vi "Sequence.ConvertColumnHeadersToChannels.vi"(8 "error in (no error)":errorcluster, 9 "Aliases.Outputs":T1[](array[typedef]), 10 "UI.Sequence#ofColumns":i32, 11 "UI.SequenceRef":refnum<vi>) -> (0 "error out":errorcluster, 1 "Warning":string, 3 "Output Channels":T1[](array[typedef]))   [LabVIEW 2015, in "Simple Sequence Tools - Editor.lvlib"]
uses:
  Simple Sequence Tools - Editor.lvlib
  Shared/Types/Channel.Properties.ctl
  Shared/SubVIs/Main.Constants.vi
  Shared/Simple Sequence Tools - Shared.lvlib
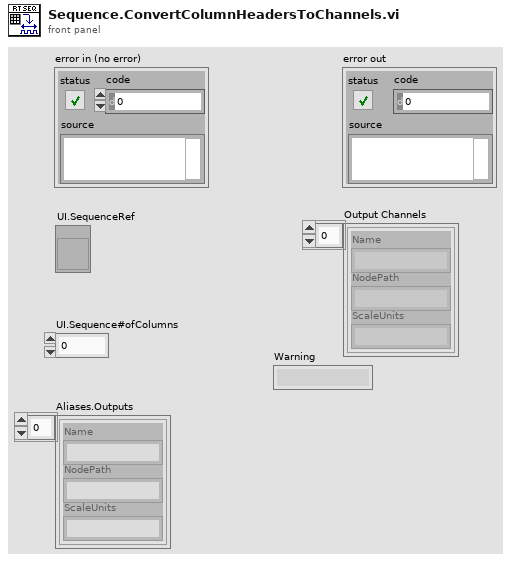
[diagram p1: front panel]
types:
  T1 = typedef "Simple Sequence Tools - Shared.lvlib/Channel.Properties.ctl" = cluster{"Name":string, "NodePath":string, "ScaleUnits":string}
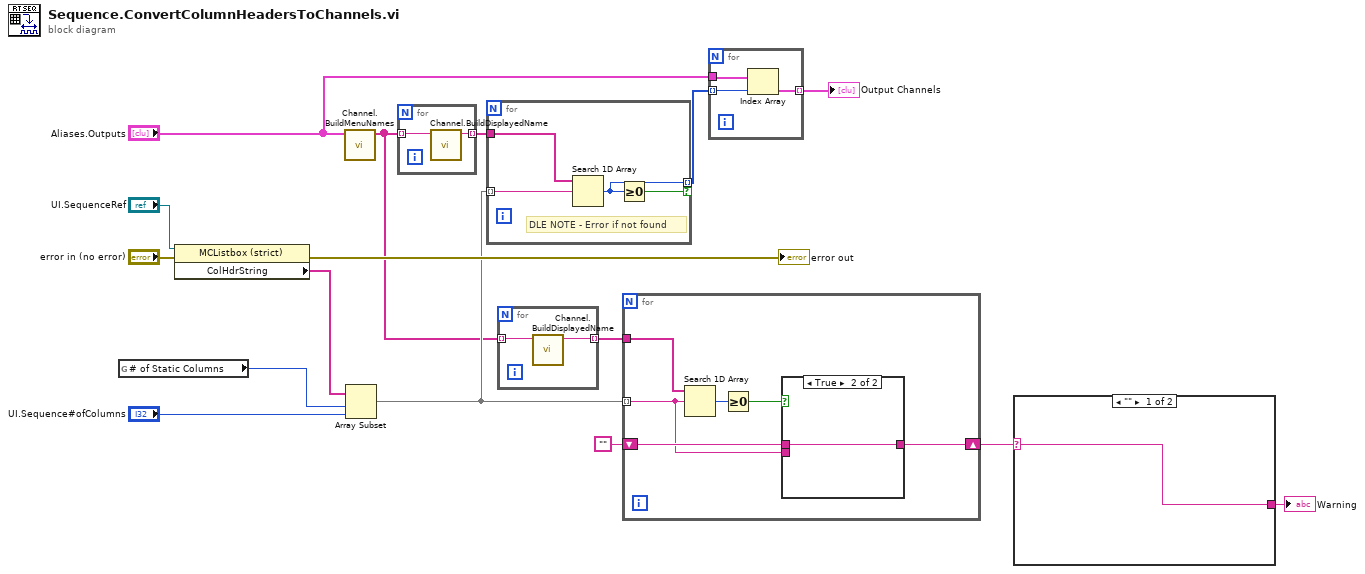
[diagram p0: block diagram]
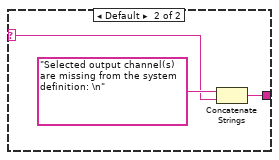
[diagram p2: hidden frame]
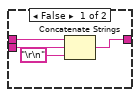
[diagram p3: hidden frame]
diagram:
  n1 = global read "Main.Constants.vi" "# of Static Columns"() -> (w3:u32)
  n2 = property class="MCListbox (strict)"(reference="UI.SequenceRef", error in="error in (no error)") -> (error out=→"error out":errorcluster, "ColHdrString"=w5:string[])  [unwired: 1 out]
  n3 = call "Channel.BuildMenuNames.vi"("Aliases"="Aliases.Outputs") -> ("Aliases Array"=w2:string[])  [unwired: 10 in]
  n4 = Array Subset(array=w5, index=w3, length="UI.Sequence#ofColumns") -> (w4:string[])
  n5 = for {
    tunnel: w2 -> [w18] mode=indexing
    tunnel: [w17] -> w1 mode=indexing
    n6 = call "Channel.BuildDisplayedName.vi"("Path"=w18) -> ("Formated Path"=w17:string)  [unwired: 10 in]
  }
  n7 = for {
    tunnel: w4 -> [w20] mode=indexing
    tunnel: [w21] -> w14 mode=indexing if=w22
    tunnel: w1 -> [w19]
    # "DLE NOTE - Error if not found"
    n8 = Search 1D Array(1D array=w19, element=w20) -> (index of element=w21:i32)  [unwired: 1 in]
    n9 = Greater Or Equal To 0?(x=w21) -> (x >= 0?=w22:bool)
  }
  n10 = for {
    tunnel: w2 -> [w24] mode=indexing
    tunnel: [w23] -> w9 mode=indexing
    n11 = call "Channel.BuildDisplayedName.vi"("Path"=w24) -> ("Formated Path"=w23:string)  [unwired: 10 in]
  }
  n12 = for {
    tunnel: w9 -> [w29]
    tunnel: w4 -> [w26] mode=indexing
    shift-right: [w27] -> w7
    shift-left: "" -> [w28]
    n13 = Search 1D Array(1D array=w29, element=w26) -> (index of element=w30:i32)  [unwired: 1 in]
    n14 = Greater Or Equal To 0?(x=w30) -> (x >= 0?=w25:bool)
    n15 = case shown="True" w25 {
      tunnel: w28 -> [w33 w35]
      tunnel: [w32 w35] -> w27
      tunnel: w26 -> [w31 _]
      frame False {
        n16 = Concatenate Strings(w33, w31, "\r\n") -> (w32:string)
      }
      frame True {
      }
    }
  }
  n17 = for {
    tunnel: w14 -> [w37] mode=indexing
    tunnel: "Aliases.Outputs" -> [w38]
    tunnel: [w36] -> w13 mode=indexing
    n18 = Index Array(array=w38, index=w37) -> (element=w36:T1)
  }
  "Output Channels" <- w13
  n19 = case shown="\"\"" w7 {
    selector: w7 -> [w39 w40]
    tunnel: [w39 w41] -> w6
    frame "" {
    }
    frame Default {
      n20 = Concatenate Strings("Selected output channel(s) are missing from the system definition: \n" ("format string"), w40) -> (w41:string)
    }
  }
  "Warning" <- w6
